vi "SelectLastUpdata.vi"(8 "error in (no error)":errorcluster, 11 "DataBase in":refnum<class "DataBase.lvclass">) -> (0 "error out":errorcluster, 2 "Data":string[][](array[string]), 3 "DataBase out":refnum<class "DataBase.lvclass">)   [LabVIEW 2019, in "DataBase.lvlib" / "DataBase.lvclass"]
uses:
  DataBase.lvclass
  DataBase.lvclass/DataBase.ctl
  <vilib>/addons/database/_DB Variant To Data/Database Variant To Data.xnode
  <vilib>/addons/database/NI_Database_API.lvlib
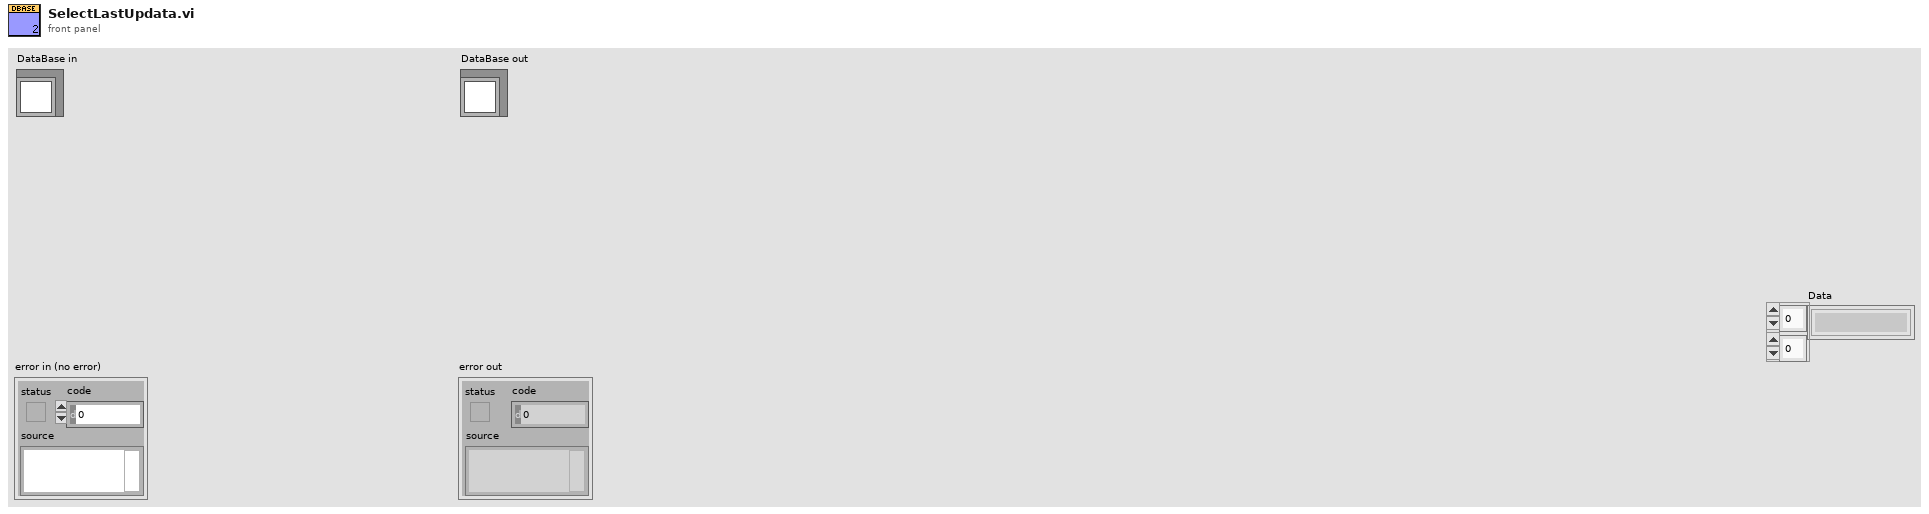
[diagram p1: front panel]
types:
  T1 = typedef "NI_Database_API.lvlib/Conn ObjectReference.ctl" = refnum<k1>
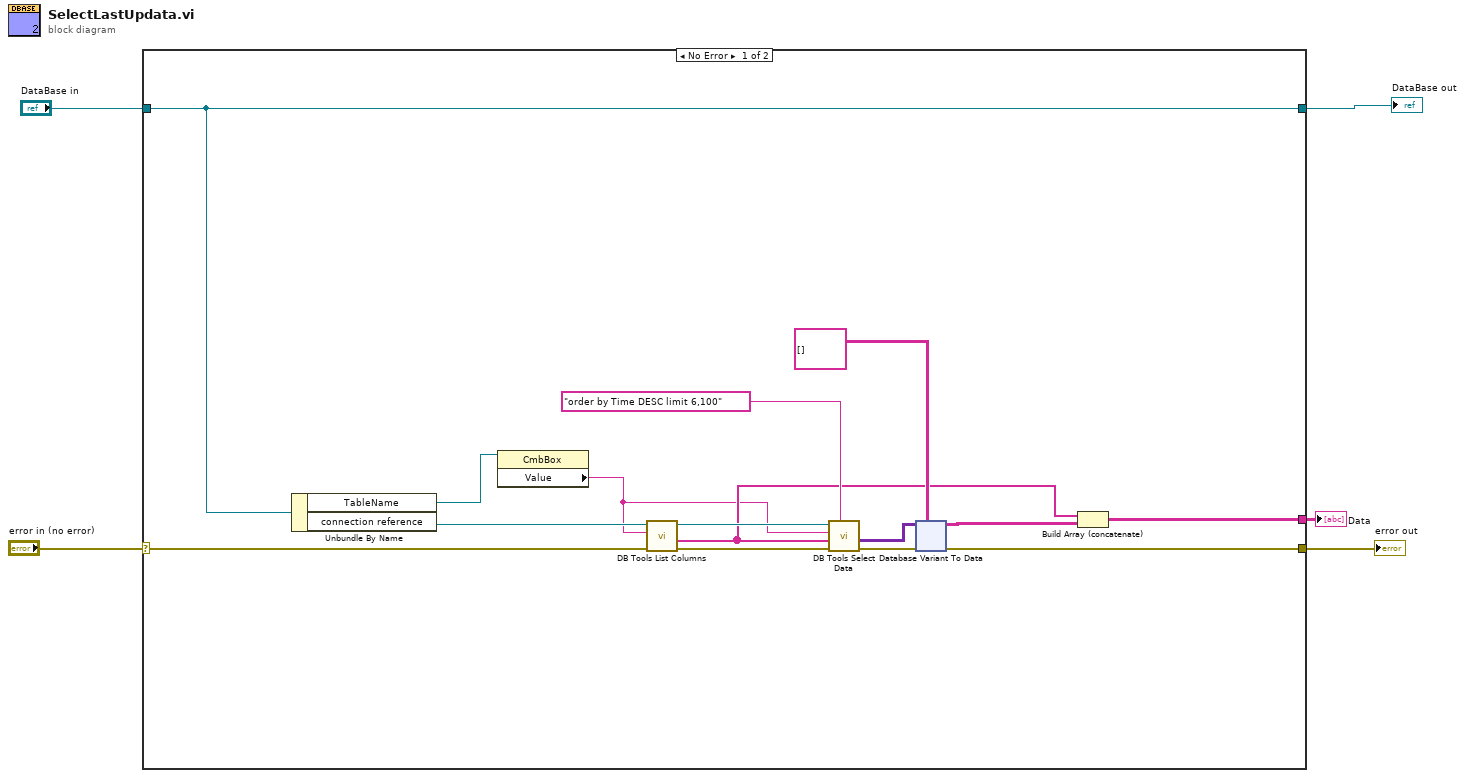
[diagram p0: block diagram]
diagram:
  n1 = case shown="No Error" "error in (no error)" {
    selector: "error in (no error)" -> [w13 w66]
    tunnel: [w11 w66] -> w4
    tunnel: [w15 w65] -> w2
    tunnel: "DataBase in" -> [w15 w65]
    tunnel: [w8 _] -> w1
    frame No Error {
      n2 = Unbundle By Name(w15) -> ("TableName"=w7:refnum<vi>, "connection reference"=w14:T1)
      n3 = property class="CmbBox"(reference=w7) -> ("Value"=w6:string)  [unwired: 1 in, 2 out]
      n4 = call <vilib>:"DB Tools List Columns.vi"("error in (no error)"=w13, "table"=w6, "connection reference"=w14) -> ("error out"=w19:errorcluster, "columns"=w9:string[], "connection reference out"=w20:T1)  [unwired: 1 in, 1 out]
      n5 = call <vilib>:"DB Tools Select Data.vi"("condition"="order by Time DESC limit 6,100", "error in (no error)"=w19, "columns"=w9, "table"=w6, "connection reference"=w20) -> ("error out"=w12:errorcluster, "data"=w17:variant[][])  [unwired: 1 in, 1 out]
      n6 = xnode "Database Variant To Data"("database variant"=w17, "error in (no error)"=w12, "type"=string[][] []) -> ("data"=w10:string[][], "error out"=w11:errorcluster)
      n7 = Build Array (concatenate)(w9, w10) -> (w8:string[][])
    }
    frame Error {
    }
  }
  "error out" <- w4
  "DataBase out" <- w2
  "Data" <- w1
